vi "GetColor.vi"(8 "error in (no error)":errorcluster, 11 "SnakeGame in":refnum<class "Snake.lvclass">) -> (0 "error out":errorcluster, 2 "Color":u32(colorbox), 3 "SnakeGame out":refnum<class "Snake.lvclass">)   [LabVIEW 2021, in "Snake.lvclass"]
uses:
  Snake.lvclass
  Snake.lvclass/Snake.ctl
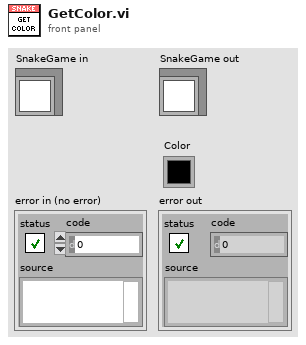
[diagram p1: front panel]
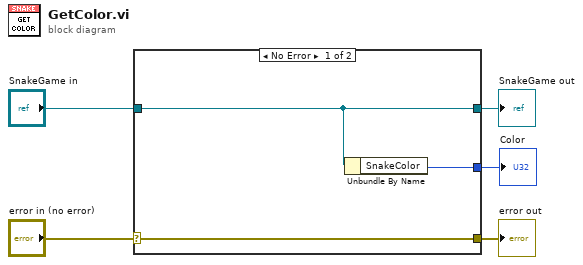
[diagram p0: block diagram]
diagram:
  n1 = case shown="No Error" "error in (no error)" {
    selector: "error in (no error)" -> [w8 w10]
    tunnel: [w8 w10] -> w4
    tunnel: [w7 w9] -> w2
    tunnel: "SnakeGame in" -> [w7 w9]
    tunnel: [w6 _] -> w1
    frame No Error {
      n2 = Unbundle By Name(w7) -> ("SnakeColor"=w6:u32)
    }
    frame Error {
    }
  }
  "error out" <- w4
  "SnakeGame out" <- w2
  "Color" <- w1
